vi "injectSample.vi"(3 "error in":errorcluster, 5 "VISA resource in":refnum<visa-resource-name>="COM10") -> (0 "error out":errorcluster, 2 "VISA resource out":refnum<visa-resource-name>="COM10")   [LabVIEW 2010]
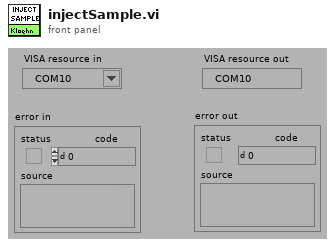
[diagram p1: front panel]
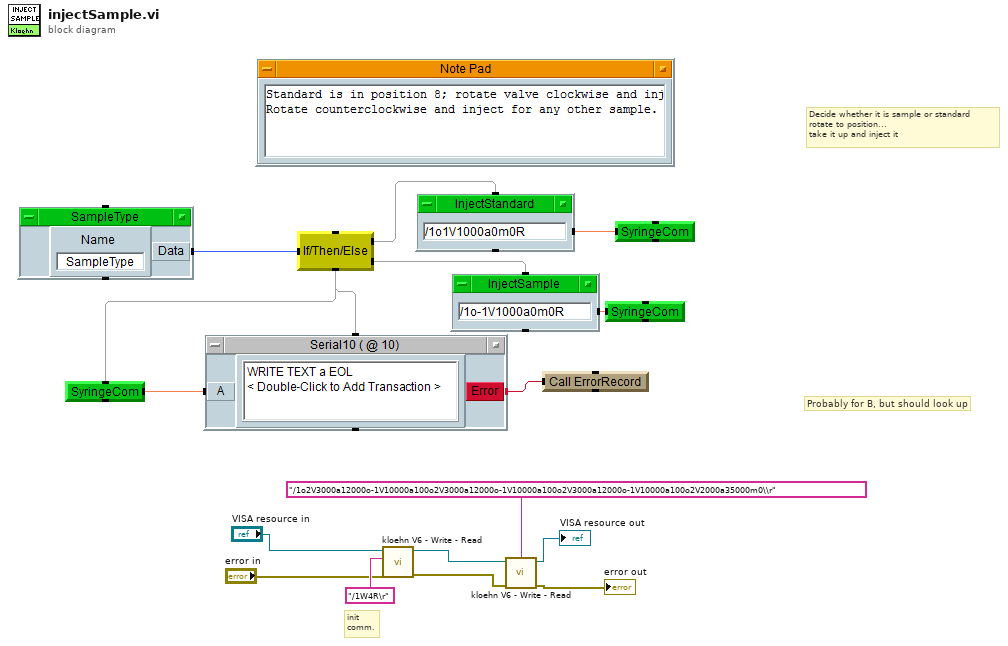
[diagram p0: block diagram]
diagram:
  # "Probably for B, but should look up"
  # "init\ncomm."
  # "Decide whether it is sample or standard\nrotate to position...\ntake it up and inject it"
  n1 = call "kloehn V6 - Write - Read.vi"("error in"="error in", "Send String"="/1W4R\r", "VISA Ref"="VISA resource in") -> ("error out"=w4:errorcluster, "VISA Ref DUP"=w5:refnum<visa-resource-name>)  [unwired: 4 in, 3 out]
  n2 = call "kloehn V6 - Write - Read.vi"("error in"=w4, "Send String"="/1o2V3000a12000o-1V10000a100o2V3000a12000o-1V10000a100o2V3000a12000o-1V10000a100o2V2000a35000m0\\r", "VISA Ref"=w5) -> ("error out"=→"error out":errorcluster, "VISA Ref DUP"=→"VISA resource out":refnum<visa-resource-name>)  [unwired: 4 in, 3 out]
